vi "TestOutputTags.vi"() -> ()   [LabVIEW 2023]
uses:
  <vilib>/ADAS Replay HIL/Channels/Tag Wrapper/Polymorphic/Open Consumer Tag (Double).vi
  <vilib>/ADAS Replay HIL/Channels/Tag Wrapper/Polymorphic/Set Default Value (Double).vi
  <vilib>/ADAS Replay HIL/Channels/Tag Wrapper/Polymorphic/Read Channel (Double).vi
  <vilib>/ADAS Replay HIL/Channels/Tag Wrapper/Polymorphic/Open Consumer Tag (Double).vi/bacb721e-673a-491a-accd-959f2e1f334e.vi
  <vilib>/ADAS Replay HIL/Channels/Tag Wrapper/Polymorphic/Set Default Value (Double).vi/228e99de-6fcf-414d-86fc-dc277c7b351f.vi
  <vilib>/ADAS Replay HIL/Channels/Tag Wrapper/Polymorphic/Read Channel (Double).vi/b2f764de-0c1e-4784-a155-687fc995a684.vi
  <vilib>/ADAS Replay HIL/Channels/Tag Wrapper/Polymorphic/Open Consumer Tag (Double).vi/bacb721e-673a-491a-accd-959f2e1f334e.vi/c28b0ead-42ad-4072-80a2-aca7f2bd7ce3.vi
  <vilib>/ADAS Replay HIL/Channels/Tag Wrapper/Polymorphic/Set Default Value (Double).vi/228e99de-6fcf-414d-86fc-dc277c7b351f.vi/4bc1c15b-36ab-481f-b8dd-c64075ce723a.vi
  <vilib>/ADAS Replay HIL/Channels/Tag Wrapper/Polymorphic/Read Channel (Double).vi/b2f764de-0c1e-4784-a155-687fc995a684.vi/c28b0ead-42ad-4072-80a2-aca7f2bd7ce3.vi
  <vilib>/ADAS Replay HIL/Channels/Tag Wrapper/Polymorphic/Read Channel (Double).vi/b2f764de-0c1e-4784-a155-687fc995a684.vi/219d0231-d98b-4193-b5cc-84f90e3c9091.vi
  <vilib>/ADAS Replay HIL/AdasHilServices/AdasHilServices Fill In Error Info Ex.vi
  <vilib>/ADAS Replay HIL/Channels/Tag Wrapper/Tag Wrapper.lvlib
  <vilib>/ADAS Replay HIL/AdasHilServices/AdasHilChannelServices.lvlib
panel:
  out "error out":errorcluster
  in  "stop":bool
  out "Power":dbl
  out "link out":errorcluster
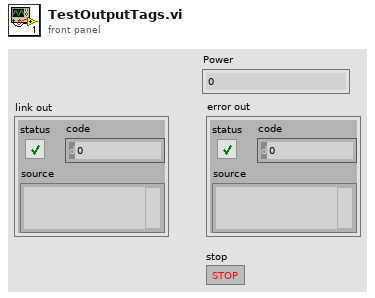
[diagram p1: front panel]
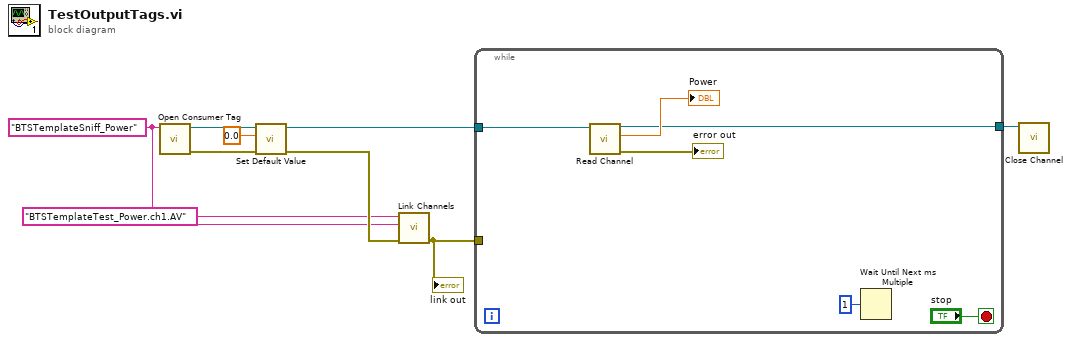
[diagram p0: block diagram]
diagram:
  w5 = "BTSTemplateSniff_Power" ("Channel Name")
  n1 = call-poly <vilib>:"Open Consumer Tag.vi"("Channel Name"=w5) -> ("error out"=w8:errorcluster, "ADAS HIL Channel"=w9:refnum<k21>)  [unwired: 9 in]
  n2 = call-poly <vilib>:"Set Default Value.vi"("error in"=w8, "Default Value"=0.0, "ADAS HIL Channel in"=w9) -> ("error out"=w6:errorcluster, "ADAS HIL Channel out"=w7:refnum<k21>)  [unwired: 7 in]
  n3 = call <vilib>:"Link Channels.vi"("error in"=w6, "Consumer Channel Name"=w5, "Producer Channel Name"="BTSTemplateTest_Power.ch1.AV") -> ("error out"=w3:errorcluster)  [unwired: 8 in]
  "link out" <- w3
  n4 = while {
    tunnel: w7 -> [w15]
    tunnel: w3 -> [_]
    tunnel: [w10] -> w2
    stop <- "stop" stop-if-true
    n5 = call-poly <vilib>:"Read Channel.vi"("ADAS HIL Channel in"=w15) -> ("error out"=→"error out":errorcluster, "Value out"=→"Power":dbl, "ADAS HIL Channel out"=w10:refnum<k21>)  [unwired: 7 in, 1 out]
    n6 = Wait Until Next ms Multiple(millisecond multiple=u32 1) -> ()  [unwired: 1 out]
  }
  n7 = call <vilib>:"Close Channel.vi"("ADAS HIL Channel"=w2) -> ()  [unwired: 10 in, 1 out]
